vi "Search_And_Delete.vi"(0 "Target_Specification_In":T1 {"Target_Address" format="%x"; "Target_Type" items=["10 Bit Address", "7 Bit Address"]}, 5 "Search_Element":string) -> (4 "Target_Specification_Out":T1 {"Target_Address" format="%x"; "Target_Type" items=["10 Bit Address", "7 Bit Address"]})   [LabVIEW 2023]
uses:
  Controls/Add_Target_Specification_.ctl
  Controls/Menu_Ring.ctl
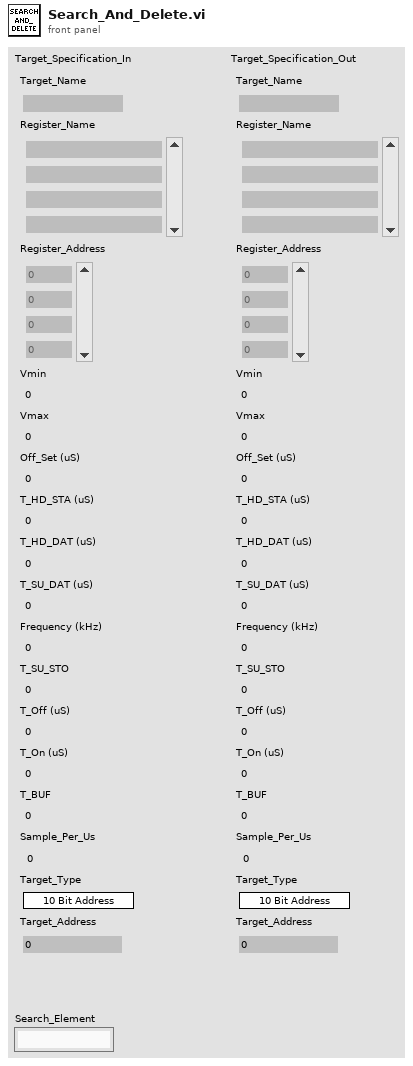
[diagram p1: front panel]
types:
  T1 = typedef "Add_Target_Specification_.ctl" = cluster{"Target_Name":string, "Register_Name":string[], "Register_Address":dbl[], "Vmin":dbl, "Vmax":dbl, "Off_Set (uS)":dbl, "T_HD_STA (uS)":dbl, "T_HD_DAT (uS)":dbl, "T_SU_DAT (uS)":dbl, "Frequency (kHz)":dbl, "T_SU_STO":dbl, "T_Off (uS)":dbl, "T_On (uS)":dbl, "T_BUF":dbl, "Sample_Per_Us":dbl, "Target_Type":T2, "Target_Address":u16}
  T2 = typedef "Menu_Ring.ctl" = u16
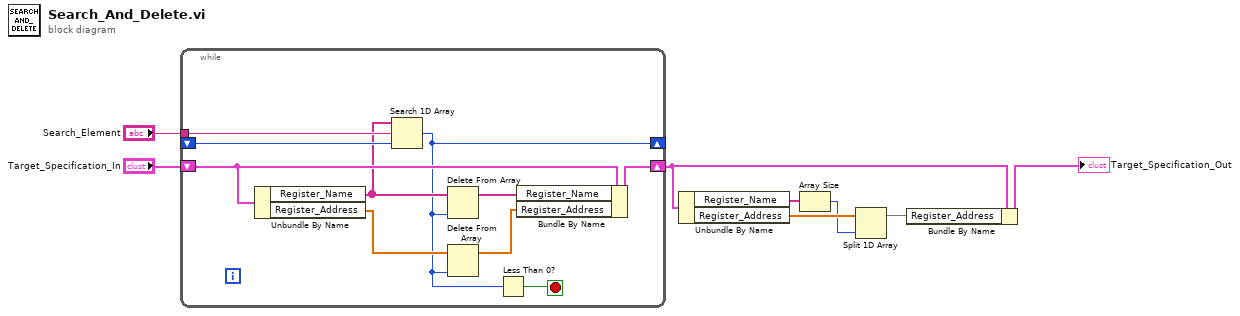
[diagram p0: block diagram]
diagram:
  n1 = while {
    tunnel: "Search_Element" -> [w18]
    shift-right: [w14] -> w6
    shift-left: "Target_Specification_In" -> [w15]
    shift-right: [w12] -> _
    shift-left: _ -> [w16]
    stop <- w11 stop-if-true
    n2 = Unbundle By Name(w15) -> ("Register_Name"=w13:string[], "Register_Address"=w17:dbl[])
    n3 = Search 1D Array(1D array=w13, element=w18, start index (0)=w16) -> (index of element=w12:i32)
    n4 = Delete From Array(array=w13, index=w12) -> (array with subset deleted=w10:string[])  [unwired: 1 in, 1 out]
    n5 = Delete From Array(array=w17, index=w12) -> (array with subset deleted=w9:dbl[])  [unwired: 1 in, 1 out]
    n6 = Less Than 0?(x=w12) -> (x < 0?=w11:bool)
    n7 = Bundle By Name(cluster=w15, "Register_Name"=w10, "Register_Address"=w9) -> (w14:T1)
  }
  n8 = Unbundle By Name(w6) -> ("Register_Name"=w4:string[], "Register_Address"=w3:dbl[])
  n9 = Array Size(array=w4) -> (size(s)=w2:i32)
  n10 = Split 1D Array(array=w3, index=w2) -> (first subarray=w1:dbl[])  [unwired: 1 out]
  n11 = Bundle By Name(cluster=w6, "Register_Address"=w1) -> (→"Target_Specification_Out":T1)
